vi "Write Style.vi"(8 "error in (no error)":errorcluster, 10 "Style":T1 items=["Modern", "Classic", "System", "NXG"], 11 "Splitter in":refnum<class "Splitter.lvclass">) -> (0 "error out":errorcluster, 3 "Splitter out":refnum<class "Splitter.lvclass">)   [LabVIEW 2020, in "Splitter.lvclass"]
uses:
  Splitter.lvclass
  Typedefs/Splitter Style--Enum.ctl
  Splitter.lvclass/Splitter.ctl
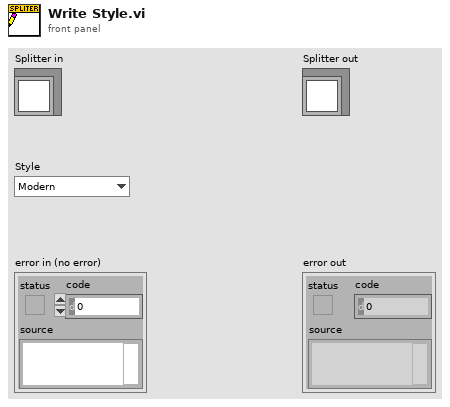
[diagram p1: front panel]
types:
  T1 = typedef "Splitter Style--Enum.ctl" = u16
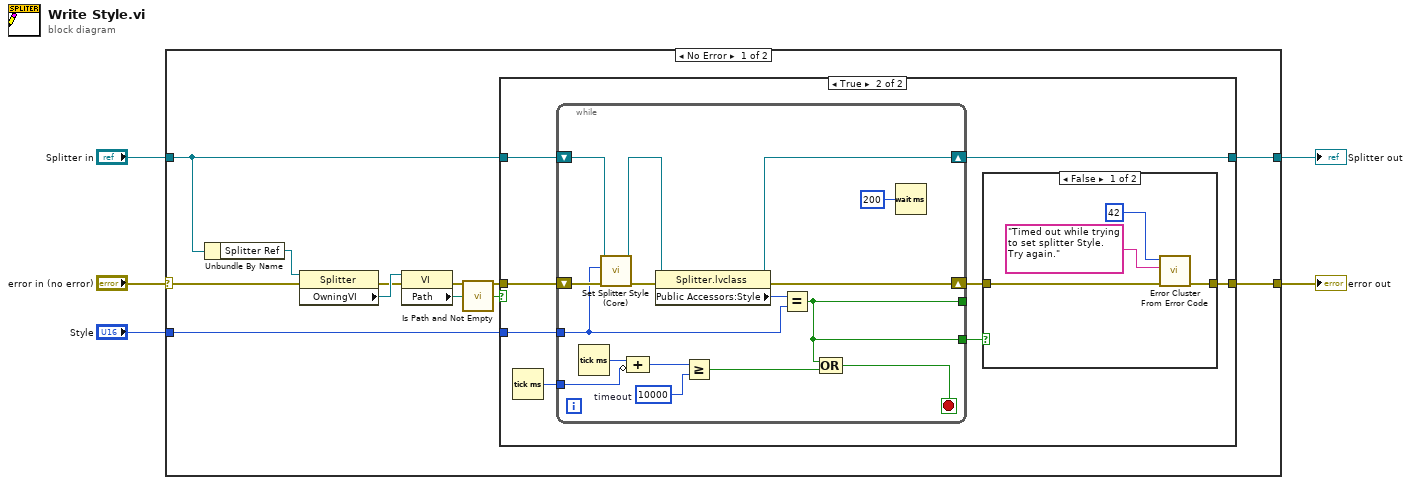
[diagram p0: block diagram]
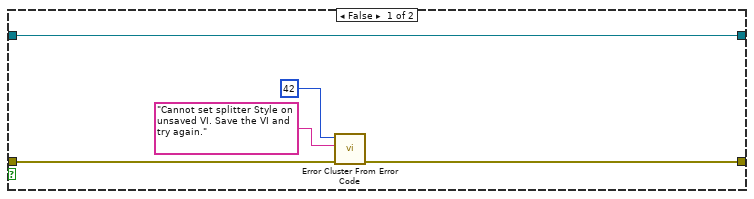
[diagram p2: hidden frame]
diagram:
  n1 = case shown="No Error" "error in (no error)" {
    selector: "error in (no error)" -> [w12 w51]
    tunnel: [w14 w51] -> w4
    tunnel: "Style" -> [w16 _]
    tunnel: "Splitter in" -> [w13 w52]
    tunnel: [w15 w52] -> w1
    frame No Error {
      n2 = Unbundle By Name(w13) -> ("Splitter Ref"=w11:refnum<vi>)
      n3 = property class="Splitter"(reference=w11, error in=w12) -> (error out=w8:errorcluster, "OwningVI"=w10:refnum<vi>)  [unwired: 1 out]
      n4 = property class="VI"(reference=w10, error in=w8) -> (error out=w9:errorcluster, "Path"=w7:path)  [unwired: 1 out]
      n5 = call <vilib>:"Is Path and Not Empty.vi"("path"=w7) -> ("Is Path and Not Empty?"=w6:bool)  [unwired: 4 in]
      n6 = case shown="True" w6 {
        tunnel: w16 -> [_ w29]
        tunnel: [w17 w28] -> w15
        tunnel: [w18 w24] -> w14
        tunnel: w13 -> [w17 w23]
        tunnel: w9 -> [w19 w22]
        frame False {
          n7 = call <vilib>:"Error Cluster From Error Code.vi"("error in (no error)"=w19, "error message (\"\")"="Cannot set splitter Style on unsaved VI. Save the VI and try again.", "error code (0)"=42) -> ("error out"=w18:errorcluster)  [unwired: 6 in]
        }
        frame True {
          n8 = Tick Count (ms)() -> (millisecond timer value=w27:u32)
          n9 = while {
            tunnel: w29 -> [w39]
            shift-right: [w30] -> w26
            shift-left: w22 -> [w45]
            shift-right: [w41] -> w28
            shift-left: w23 -> [w43]
            tunnel: w27 -> [w36]
            tunnel: [w32] -> _
            tunnel: [w32] -> w25
            stop <- w38 stop-if-true
            w34 = u32 10000  # timeout
            n10 = Tick Count (ms)() -> (millisecond timer value=w37:u32)
            n11 = call "Set Splitter Style (Core).vi"("error in (no error)"=w45, "Style"=w39, "Splitter in"=w43) -> ("error out"=w44:errorcluster, "Splitter out"=w42:refnum<class "Splitter.lvclass">)  [unwired: 7 in]
            n12 = Compound Arithmetic op=ADD(w37, invert w36) -> (w35:u32)
            n13 = property class="Splitter.lvclass"(reference=w42, error in=w44) -> (reference out=w41:refnum<class "Splitter.lvclass">, error out=w30:errorcluster, "Public Accessors:Style"=w40:T1)
            n14 = Greater Or Equal?(x=w35, y=w34) -> (x >= y?=w33:bool)
            n15 = Equal?(x=w40, y=w39) -> (x = y?=w32:bool)
            n16 = Compound Arithmetic op=OR(w32, w33) -> (w38:bool)
            n17 = Wait (ms)(milliseconds to wait=u32 200) -> ()  [unwired: 1 out]
          }
          n18 = case shown="False" w25 {
            tunnel: w26 -> [w49 w50]
            tunnel: [w48 w50] -> w24
            frame False {
              n19 = call <vilib>:"Error Cluster From Error Code.vi"("error in (no error)"=w49, "error message (\"\")"="Timed out while trying to set splitter Style. Try again.", "error code (0)"=42) -> ("error out"=w48:errorcluster)  [unwired: 6 in]
            }
            frame True {
            }
          }
        }
      }
    }
    frame Error {
    }
  }
  "error out" <- w4
  "Splitter out" <- w1
